vi "svfa_Process Coherence (complex).vi"(0 "X FFT spectrum [Vrms]":cluster{"f0":dbl, "df":dbl, "spectrum":cdb[]} {"spectrum" format="%.2f"; "df" format="%.2f"; "f0" format="%.2f"}, 1 "processing control":T1(ring), 7 "Y FFT spectrum [Vrms]":cluster{"f0":dbl, "df":dbl, "spectrum":cdb[]} {"spectrum" format="%.2f"; "df" format="%.2f"; "f0" format="%.2f"}, 9 "averaging parameters":T2={"averaging mode"=enum."No averaging", "weighting mode"=enum."Linear", "number of averages"=10, "linear mode"=enum."Auto restart"}, 11 "error in (no error)":errorcluster) -> (2 "averaging done":bool, 3 "averages completed":dbl format="%.2f", 4 "Coherence":dbl[](array[numeric]) format="%.2f", 6 "MAG <Gxy>":dbl[](array[numeric]) format="%.2f", 8 "<Gxx>":dbl[](array[numeric]) format="%.2f", 10 "<Gyy>":dbl[](array[numeric]) format="%.2f", 14 "PHASE <Gxy>":dbl[](array[numeric]) format="%.2f", 15 "error out":errorcluster)   [LabVIEW 2017]
uses:
  <vilib>/addons/_NISVFA/_Shared subVIs/Spectrum Averaging/svfa_Average Array with Avg Checks (real) No State.vi
  <vilib>/addons/_NISVFA/_Shared subVIs/Spectrum Averaging/svfa_Reset Averaging State Info.vi
  <vilib>/addons/_NISVFA/_Shared subVIs/Spectrum Averaging/svfa_Average Array with Avg Checks (complex) No State.vi
  <vilib>/addons/_NISVFA/_Shared subVIs/Spectrum Averaging/svfa_Average Array (real) No State.vi
  <vilib>/addons/_NISVFA/_Shared subVIs/Spectrum Averaging/svfa_Average Array (complex) No State.vi
  <vilib>/addons/_NISVFA/_Shared subVIs/Spectrum Averaging/svfa_No Average Array (real).vi
  <vilib>/addons/_NISVFA/_Shared subVIs/Spectrum Averaging/svfa_Average Array (real).vi
  <vilib>/addons/_NISVFA/_Shared subVIs/Spectrum Averaging/svfa_Peak Hold Array.vi
  <vilib>/addons/_NISVFA/_Shared subVIs/Spectrum Averaging/svfa_No Average Array (complex).vi
  <vilib>/addons/_NISVFA/_Shared subVIs/Spectrum Averaging/svfa_Average Array (complex).vi
panel:
  out "df":dbl format="%.2f"
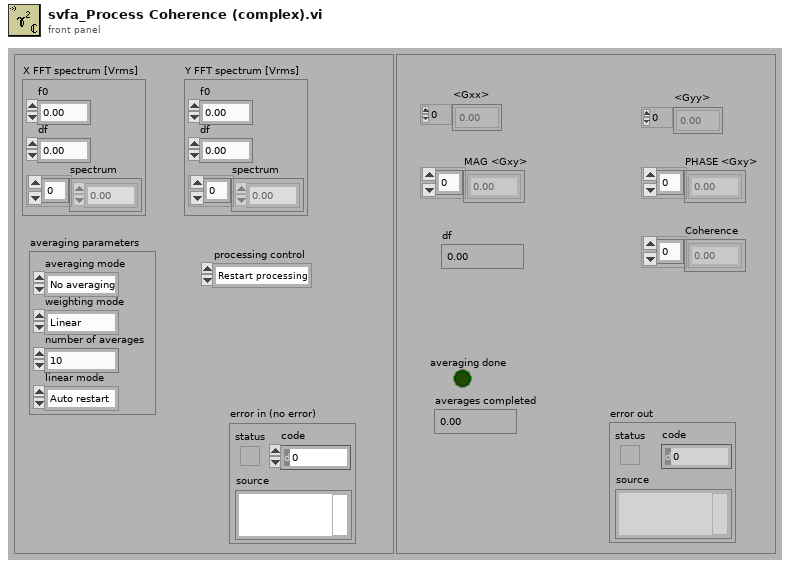
[diagram p1: front panel]
types:
  T1 = enum16{"Restart processing", "Continue processing", "Skip processing"}
  T2 = cluster{"averaging mode":enum16{"No averaging", "Vector averaging", "RMS averaging", "Peak hold"}, "weighting mode":enum16{"Linear", "Exponential"}, "number of averages":u32, "linear mode":enum16{"One shot", "Auto restart"}}
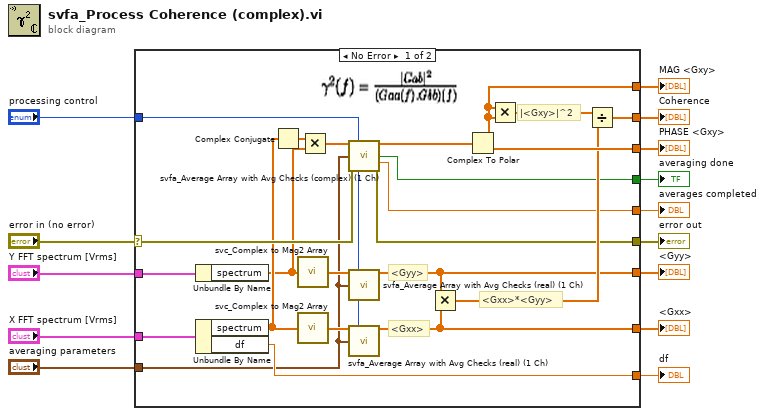
[diagram p0: block diagram]
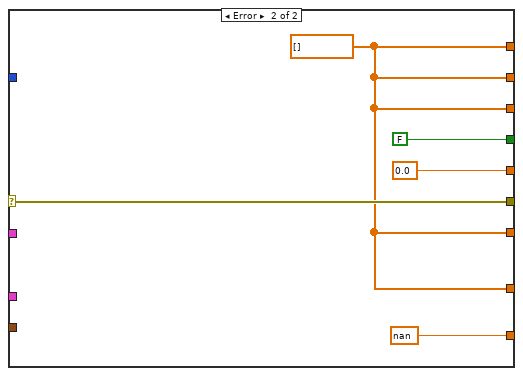
[diagram p2: hidden frame]
diagram:
  n1 = case shown="No Error" "error in (no error)" {
    selector: "error in (no error)" -> [w29 w42]
    tunnel: [w36 w41] -> w14
    tunnel: [w35 w41] -> w13
    tunnel: "X FFT spectrum [Vrms]" -> [w23 _]
    tunnel: "averaging parameters" -> [w15 _]
    tunnel: [w25 w41] -> w10
    tunnel: "processing control" -> [w32 _]
    tunnel: [w34 w41] -> w8
    tunnel: [w16 nan ("df")] -> w7
    tunnel: [w30 FALSE ("averaging done")] -> w6
    tunnel: [w31 0.0 ("averages completed")] -> w5
    tunnel: [w27 w42] -> w4
    tunnel: [w26 w41] -> w3
    tunnel: "Y FFT spectrum [Vrms]" -> [w24 _]
    frame No Error {
      # "<Gyy>"
      # "<Gxx>"
      # "<Gxx>*<Gyy>"
      # "|<Gxy>|^2"
      n2 = Unbundle By Name(w24) -> ("spectrum"=w17:cdb[])
      n3 = Unbundle By Name(w23) -> ("spectrum"=w18:cdb[], "df"=w16:dbl)
      n4 = Complex Conjugate(1:w18) -> (0:w22:cdb[])
      n5 = call <vilib>:"svc_Complex to Mag2 Array.vi"("complex array"=w17) -> ("magnitude^2 array"=w19:dbl[])  [unwired: 4 in]
      n6 = call <vilib>:"svc_Complex to Mag2 Array.vi"("complex array"=w18) -> ("magnitude^2 array"=w20:dbl[])  [unwired: 4 in]
      n7 = Multiply(x=w22, y=w17) -> (x*y=w21:cdb[])
      n8 = call <vilib>:"svfa_Average Array with Avg Checks (complex) (1 Ch).vi"("spectrum"=w21, "processing control"=w32, "averaging parameters"=w15, "error in (no error)"=w29) -> ("average spectrum"=w28:cdb[], "averaging done"=w30:bool, "averages completed"=w31:dbl, "error out"=w27:errorcluster)  [unwired: 7 in, 1 out]
      n9 = call <vilib>:"svfa_Average Array with Avg Checks (real) (1 Ch).vi"("spectrum"=w19, "processing control"=w32, "averaging parameters"=w15) -> ("average spectrum"=w26:dbl[])  [unwired: 8 in, 4 out]
      n10 = call <vilib>:"svfa_Average Array with Avg Checks (real) (1 Ch).vi"("spectrum"=w20, "processing control"=w32, "averaging parameters"=w15) -> ("average spectrum"=w25:dbl[])  [unwired: 8 in, 4 out]
      n11 = Multiply(x=w26, y=w25) -> (x*y=w33:dbl[])
      n12 = Complex To Polar(r * e^(i*theta)=w28) -> (r=w35:dbl[], theta=w34:dbl[])
      n13 = Multiply(x=w35, y=w35) -> (x*y=w37:dbl[])
      n14 = Divide(x=w37, y=w33) -> (x/y=w36:dbl[])
    }
    frame Error {
      w41 = dbl[] []
    }
  }
  "Coherence" <- w14
  "<Gxx>" <- w10
  "<Gyy>" <- w3
  "MAG <Gxy>" <- w13
  "PHASE <Gxy>" <- w8
  "averages completed" <- w5
  "error out" <- w4
  "averaging done" <- w6
  "df" <- w7
